vi "Elevator State Control.vi"() -> ()   [LabVIEW 2018]
uses:
  RefNumsDriverStation.vi
  Users/marka/Desktop/Secret City Wildbots Summer Project/2019_Robot_Project/2019 Summer Rebuild/Sensor Readings.vi
panel:
  out "Target_Vacuum_Pump_Power":dbl
  out "Target_Elevator_Position":dbl
  out "Elevator_State_Out":string
  in  "Elevator_State":string
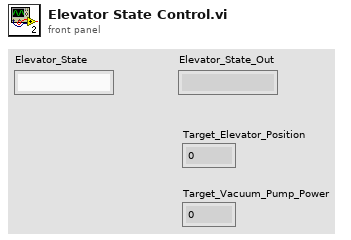
[diagram p1: front panel]
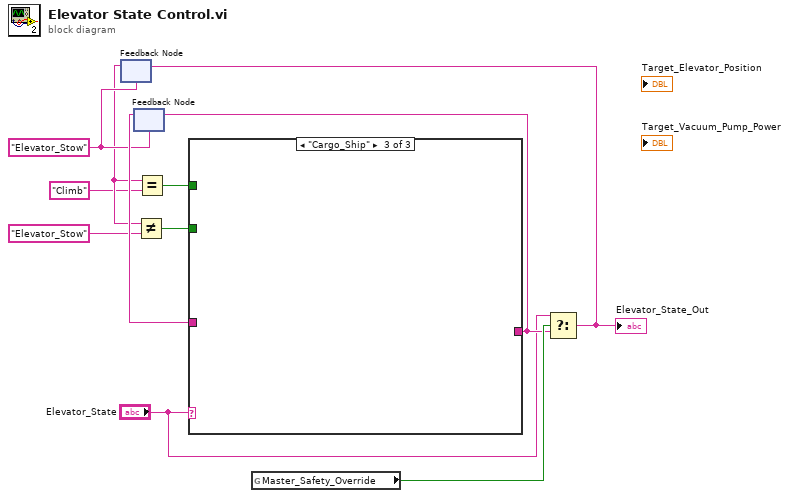
[diagram p0: block diagram]
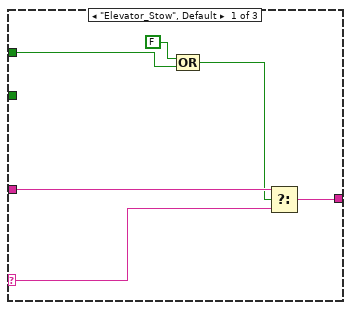
[diagram p2: hidden frame]
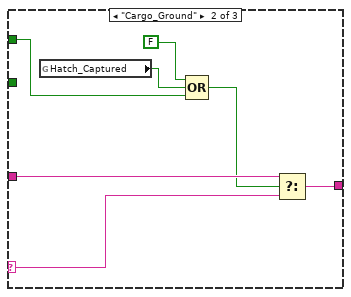
[diagram p3: hidden frame]
diagram:
  w7 = "Elevator_Stow" ("Elevator_State")
  n1 = feedback #1(w7) -> (w5:string)
  n2 = feedback #2(w7) -> (w10:string)
  n3 = Not Equal?(x=w5, y="Elevator_Stow") -> (x != y?=w3:bool)
  n4 = Equal?(x=w5, y="Climb") -> (x = y?=w2:bool)
  n5 = case shown="\"Cargo_Ship\"" "Elevator_State" {
    selector: "Elevator_State" -> [w12 w20 _]
    tunnel: [w17 w21 _] -> w9
    tunnel: w10 -> [w16 w19 _]
    tunnel: w3 -> [_ _ _]
    tunnel: w2 -> [w15 w24 _]
    frame "Elevator_Stow", Default {
      n6 = Compound Arithmetic op=OR(FALSE ("value"), w15) -> (w13:bool)
      n7 = Select(t=w16, s=w13, f=w12) -> (s? t:f=w17:string)
    }
    frame "Cargo_Ground" {
      n8 = global read "Sensor Readings.vi" "Hatch_Captured"() -> (w23:bool)
      n9 = Compound Arithmetic op=OR(FALSE ("value"), w23, w24) -> (w18:bool)
      n10 = Select(t=w19, s=w18, f=w20) -> (s? t:f=w21:string)
    }
    frame "Cargo_Ship" {
    }
  }
  n11 = feedback-in #2(w9) -> ()
  n12 = global read "RefNumsDriverStation.vi" "Master_Safety_Override"() -> (w11:bool)
  n13 = Select(t="Elevator_State", s=w11, f=w9) -> (s? t:f=w8:string)
  "Elevator_State_Out" <- w8
  n14 = feedback-in #1(w8) -> ()
